vi "Initialize Hardware.vi"(8 "error in (no error)":errorcluster, 9 "DAQ Type":enum16{"Hardware", "Simulation"}(ring), 10 "Connection Setting":T1={"Ref"=variant, "Serial"={"Baud Rate"=9600, "Parity"=0, "Data Bits"=8, "Flow Control"=4}} {"Serial"."Flow Control" items=["None", "XON/XOFF", "RTS/CTS", "XON/XOFF & RTS/CTS", "DTR/DSR", "XON/XOFF & DTR/DSR"]; "Serial"."Data Bits" items=["7"=7, "8"=8]; "Serial"."Parity" items=["None", "Odd", "Even", "Mark", "Space"]; "Serial"."Baud Rate" items=["300"=300, "600"=600, "1200"=1200, "2400"=2400, "4800"=4800, "9600"=9600, "19200"=19200]}, 11 "Abstract in":refnum<class "Abstract.lvclass">) -> (0 "error out":errorcluster, 3 "Abstract out":refnum<class "Abstract.lvclass">)   [LabVIEW 2016, in "Func Generator.lvlib" / "Abstract.lvclass"]
uses:
  Abstract.lvclass
  Instrument Setting.ctl
  Func Generator.lvlib
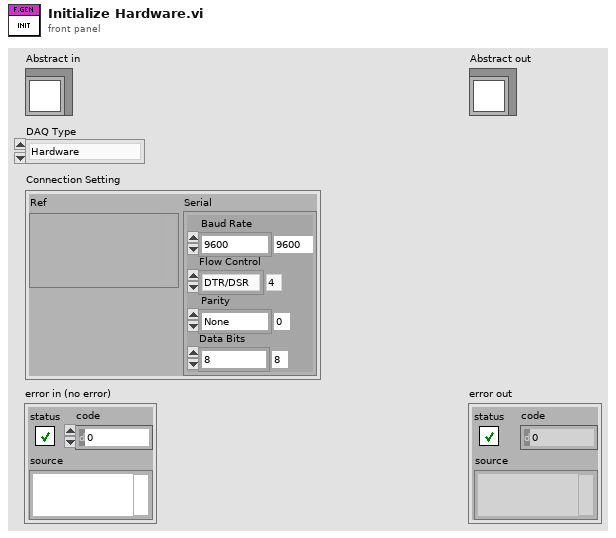
[diagram p1: front panel]
types:
  T1 = typedef "Func Generator.lvlib/Instrument Setting.ctl" = cluster{"Ref":variant, "Serial":cluster{"Baud Rate":u32, "Parity":u16, "Data Bits":u16, "Flow Control":u16}}
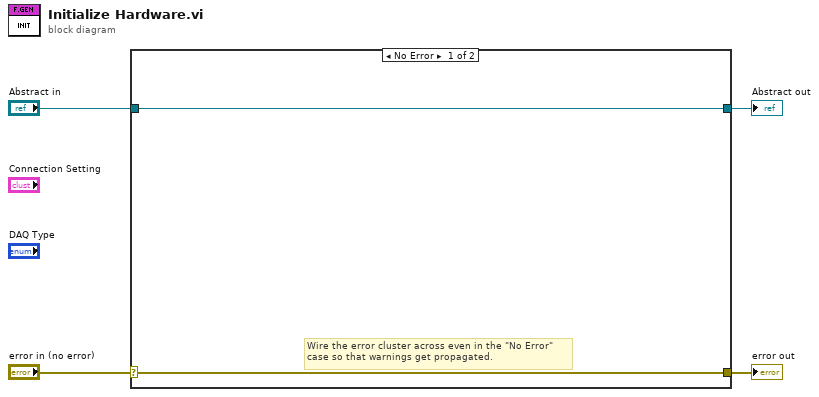
[diagram p0: block diagram]
diagram:
  n1 = case shown="No Error" "error in (no error)" {
    selector: "error in (no error)" -> [w5 w8]
    tunnel: [w5 w8] -> w3
    tunnel: [w6 w7] -> w1
    tunnel: "Abstract in" -> [w6 w7]
    frame No Error {
      # "Wire the error cluster across even in the \"No Error\"\ncase so that warnings get propagated."
    }
    frame Error {
    }
  }
  "error out" <- w3
  "Abstract out" <- w1
